vi "Create Linear Vector by Step.vi"(8 "error in (no error)":errorcluster, 9 "Step":dbl, 10 "Stop":dbl, 11 "Start":dbl) -> (0 "error out":errorcluster, 2 "Count":i32, 3 "Vector":dbl[](array[numeric]))   [LabVIEW 2019]
uses:
  <vilib>/Analysis/1siggen.llb/Ramp Pattern by Delta.vi
  <vilib>/Analysis/NI_AALBase.lvlib
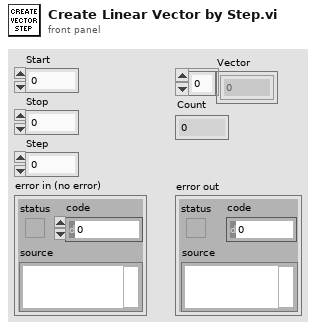
[diagram p1: front panel]
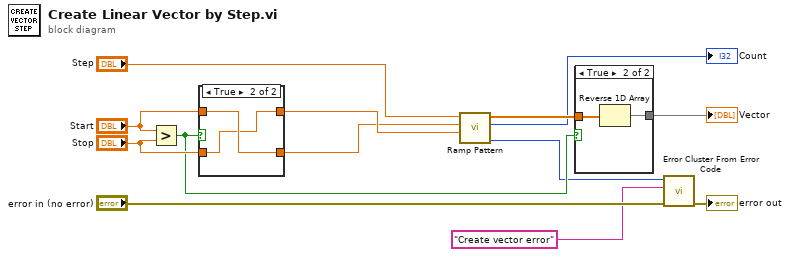
[diagram p0: block diagram]
diagram:
  n1 = Greater?(x="Start", y="Stop") -> (0:w7:bool)
  n2 = case shown="True" w7 {
    tunnel: "Start" -> [w15 w17]
    tunnel: "Stop" -> [w14 w16]
    tunnel: [w15 w16] -> w11
    tunnel: [w14 w17] -> w10
    frame False {
    }
    frame True {
    }
  }
  n3 = call-poly <vilib>:"Ramp Pattern.vi"("start"=w11, "end"=w10, "delta"="Step") -> ("error"=w4:i32, "samples"=→"Count":i32, "Ramp Pattern"=w8:dbl[])  [unwired: 6 in]
  n4 = case shown="True" w7 {
    tunnel: w8 -> [w18 w20]
    tunnel: [w18 w19] -> w6
    frame False {
    }
    frame True {
      n5 = Reverse 1D Array(array=w20) -> (reversed array=w19:dbl[])
    }
  }
  "Vector" <- w6
  n6 = call <vilib>:"Error Cluster From Error Code.vi"("error in (no error)"="error in (no error)", "error message (\"\")"="Create vector error" ("error message (\"\")"), "error code (0)"=w4) -> ("error out"=→"error out":errorcluster)  [unwired: 6 in]
